vi "WriteBytes.vi"(8 "error in (no error)":errorcluster, 10 "Data":u8[](array[numeric]), 11 "mainI2CDevice in":refnum<class "mainI2CDevice.lvclass">) -> (0 "error out":errorcluster, 3 "mainI2CDevice out":refnum<class "mainI2CDevice.lvclass">)   [LabVIEW 2020, in "RPI.lvlib" / "mainI2CDevice.lvclass"]
doc: "Write data bytes to the I2C slave device."
uses:
  mainI2CDevice.lvclass
  mainI2CDevice.lvclass/mainI2CDevice.ctl
  <vilib>/MakerHub/LINX/Private/Local IO/LinxI2cWrite.vi
  <vilib>/MakerHub/LINX/Public/Utilities/Check Channel.vi
  <vilib>/MakerHub/LINX/Private/Local IO/Handle Errors.vi
  <vilib>/MakerHub/LINX/Private/Utilties/Generate Error.vi
  <vilib>/MakerHub/LINX/LMH-LINX.lvlib
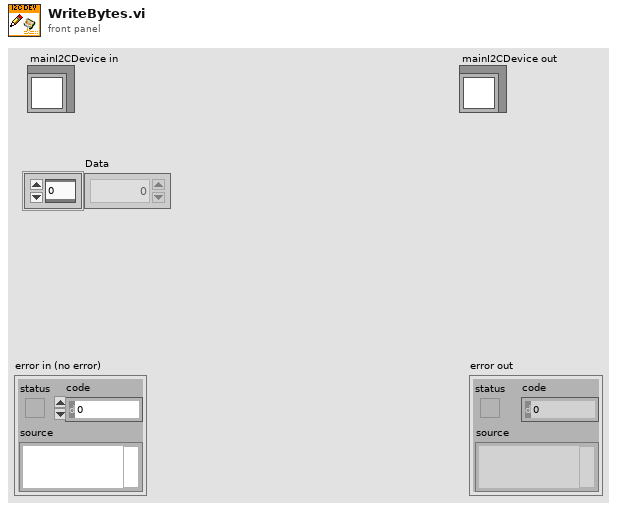
[diagram p1: front panel]
types:
  T1 = typedef "LMH-LINX.lvlib/LINX Ref.ctl" = cluster{"IO":T2, "Interface":T3, "LINX Device Config":T4}
  T2 = typedef "LMH-LINX.lvlib/Platform.ctl" = enum16{"Remote", "Local"}
  T3 = typedef "LMH-LINX.lvlib/Interface.ctl" = enum16{"Serial", "TCP"}
  T4 = typedef "LMH-LINX.lvlib/Device.lvlib/LINX Device Config.ctl" = cluster{"Interface":T3, "COM Port":refnum<visa-resource-name>, "TCP Configuration":T5, "Device Family":u8, "Device ID":u8, "Device Name":string, "TCP Ref":refnum<k5>, "Channels":T6}
  T5 = typedef "LMH-LINX.lvlib/Device.lvlib/TCP Config.ctl" = cluster{"IP Address":string, "Port":u16}
  T6 = typedef "LMH-LINX.lvlib/Channels.ctl" = cluster{"DI":u8[], "DO":u8[], "AI":u8[], "AO":u8[], "PWM":u8[], "QE":u8[], "UART":u8[], "I2C 2":u8[], "SPI":u8[], "CAN":u8[], "Servo":u8[], "AI Ref (V)":dbl, "AI Resolution (Bits)":u8, "AO Ref (V)":dbl, "AO Resolution (Bits)":u8}
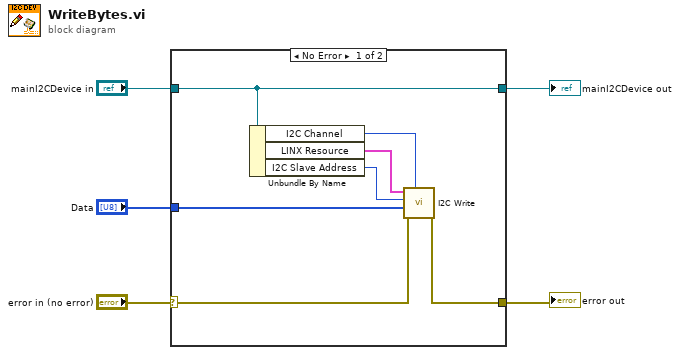
[diagram p0: block diagram]
diagram:
  n1 = case shown="No Error" "error in (no error)" {
    selector: "error in (no error)" -> [w7 w14]
    tunnel: [w6 w14] -> w4
    tunnel: [w11 w13] -> w2
    tunnel: "mainI2CDevice in" -> [w11 w13]
    tunnel: "Data" -> [w8 _]
    frame No Error {
      n2 = Unbundle By Name(w11) -> ("I2C Channel"=w9:u8, "LINX Resource"=w12:T1, "I2C Slave Address"=w10:u8)
      n3 = call <vilib>:"I2C Write.vi"("I2C Channel"=w9, "Error In"=w7, "Data"=w8, "I2C Slave Address (0)"=w10, "LINX Resource"=w12) -> ("Error Out"=w6:errorcluster)  [unwired: 5 in, 1 out]
    }
    frame Error {
    }
  }
  "error out" <- w4
  "mainI2CDevice out" <- w2
